vi "RollingCurrentReadout.vi"(4 "settling\ndelay":i32, 6 "Base/High Voltage?":enum16{"Base voltage", "High voltage"}(ring), 7 "Current Threshold [nA]":dbl, 8 "disabled channels IN":i32[](array[numeric]), 9 "Flag IN":i32[](array[numeric]), 10 "Current Array IN [nA]":dbl[](array[numeric])) -> (0 "disabled channels OUT":i32[](array[numeric]), 1 "Flag OUT":i32[](array[numeric]), 3 "Current Array OUT [nA]":dbl[](array[numeric]), 5 "Compliance exceeded":bool)   [LabVIEW 2013]
doc: "Switching through channels connected to a Probe Card"
uses:
  InstrControl/SupplyControl/SupplyControl.lvclass
  general_VIs/globals/QC_MeasurementSetup.vi
  InstrControl/InstrumentSetup.vi
  InstrControl/Switching/Switching.lvclass
  InstrControl/InstrControl.lvclass
panel:
  out "Display MUX":bool[][](array[boolean])
  out "Pinhole Flag":i32
  in  "last channel completed":i32
  # "Pickering Multiplexer Settings"
  # "X1"
  # "X2"
  # "X3"
  # "X4"
  # "X5"
  # "X6"
  # "X7"
  # "X8"
  # "Y1  Y2  Y3  Y4"
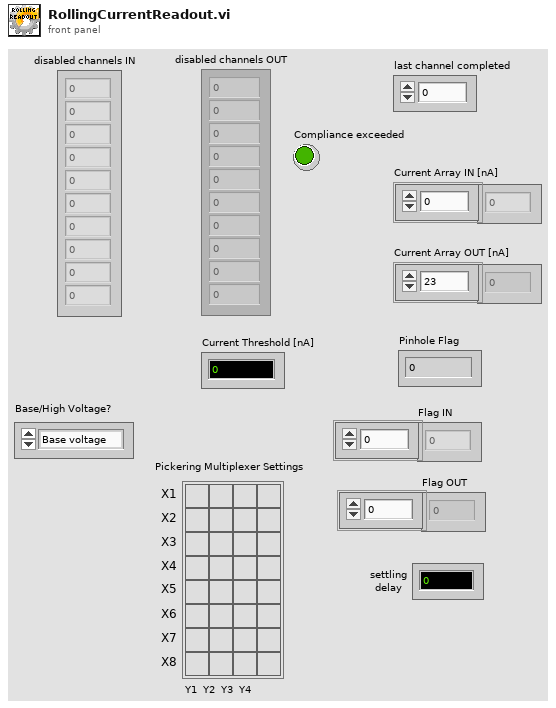
[diagram p1: front panel]
types:
  T1 = cluster{"Bias Supply":refnum<class "SupplyControl.lvclass">, "SMU":refnum<class "SupplyControl.lvclass">, "LCR":refnum<class "LCRControl.lvclass">, "Probe Card Channels":i32, "Bias Voltage [V]":dbl, "First strip":i32, "Last strip":i32, "Base Voltage [V]":dbl, "Base Ramp Step [V]":dbl, "Base Ramp Interval [ms]":u32, "High Voltage [V]":dbl, "High Ramp Step [V]":dbl, "High Ramp Interval [ms]":u32, "Single Needle":bool, "ArduinoControl.lvclass":refnum<class "ArduinoControl.lvclass">, "Fraction of good strips [%]":dbl}
  T2 = cluster{"GPIB address":string, "Matrix address":string, "Mux1 address":string, "Mux2 address":string, "Matrix used?":bool, "Switching":refnum<class "Switching.lvclass">, "Matrix X Channels":cluster{"Bias Supply / SMU LO":i32, "Bias Supply / SMU HI":i32, "CV Box LO":i32, "CV Box HI":i32, "CV Box LO IN":i32, "CV Box HI IN":i32, "Volt meter LO":i32, "Volt meter HI":i32, "Mux1 C1":i32, "Mux1 C2":i32, "Mux2 C1":i32, "Mux2 C2":i32}}
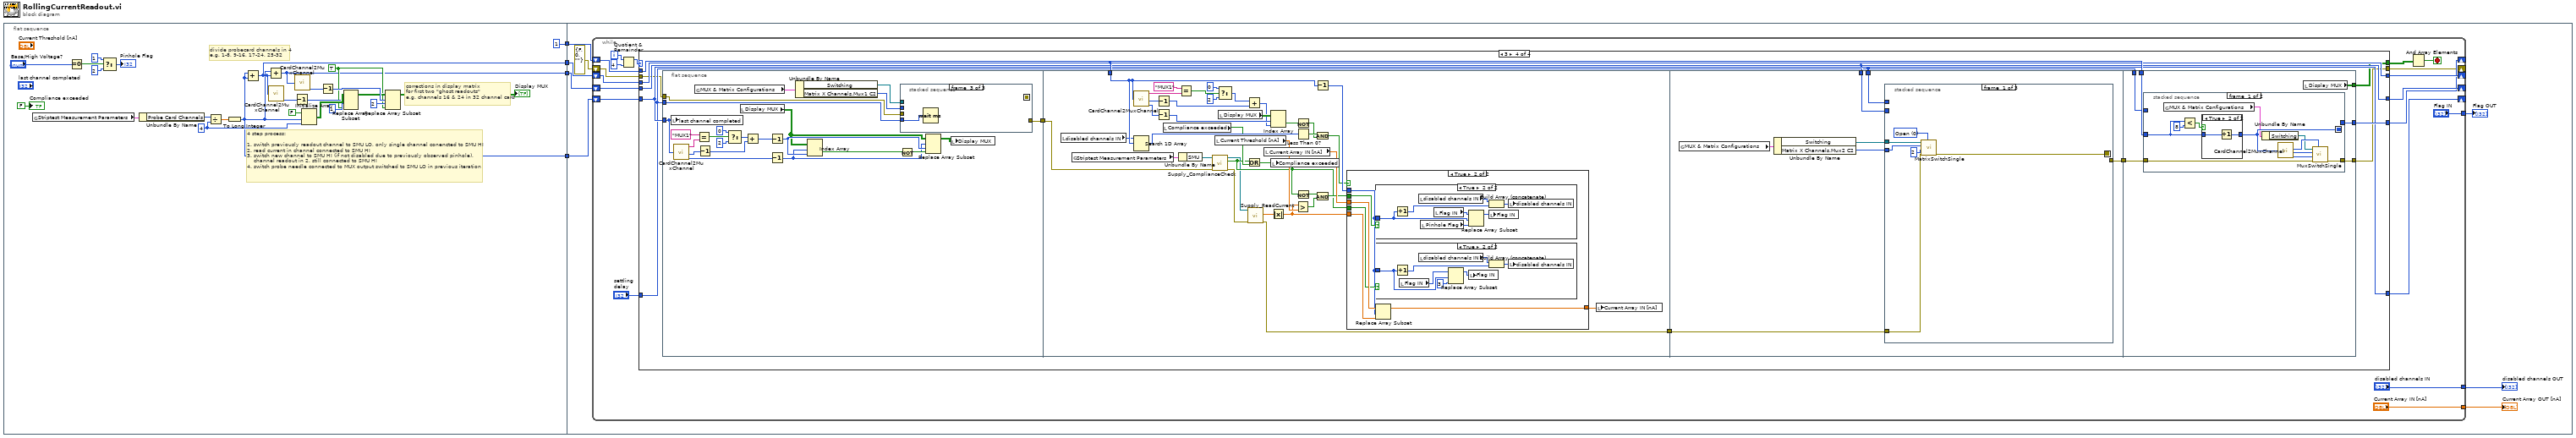
[diagram p0: block diagram]
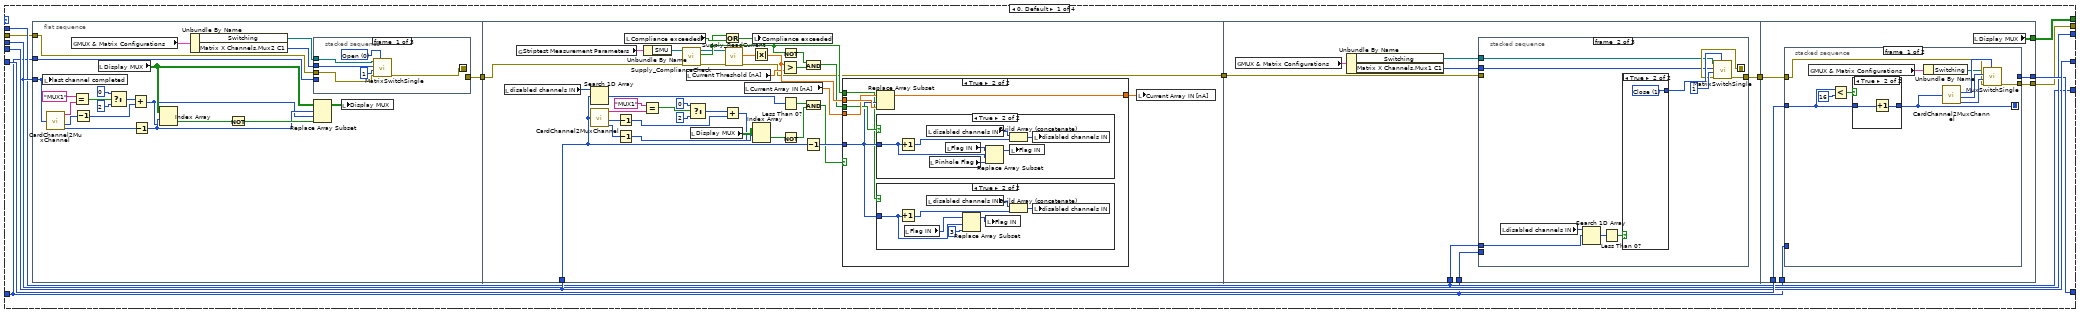
[diagram p2: hidden frame]
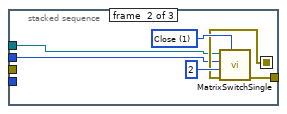
[diagram p3: hidden frame]
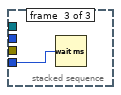
[diagram p4: hidden frame]
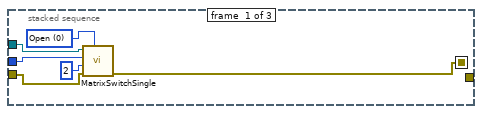
[diagram p8: hidden frame]
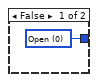
[diagram p9: hidden frame]
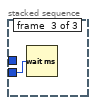
[diagram p10: hidden frame]
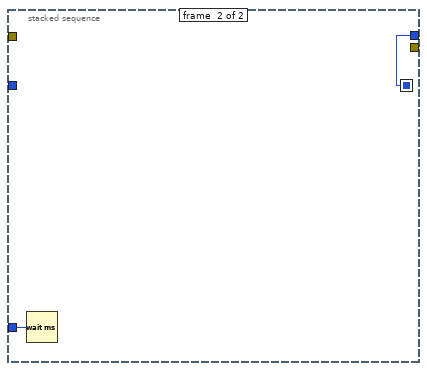
[diagram p12: hidden frame]
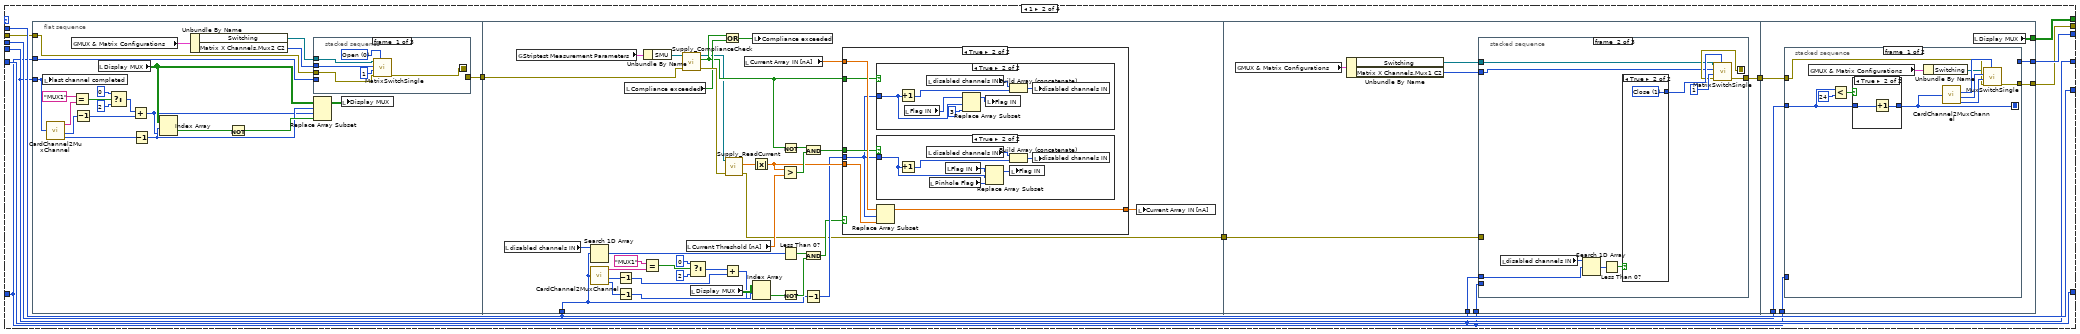
[diagram p13: hidden frame]
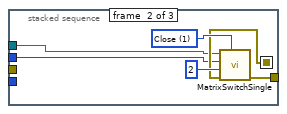
[diagram p14: hidden frame]
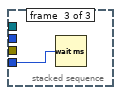
[diagram p15: hidden frame]
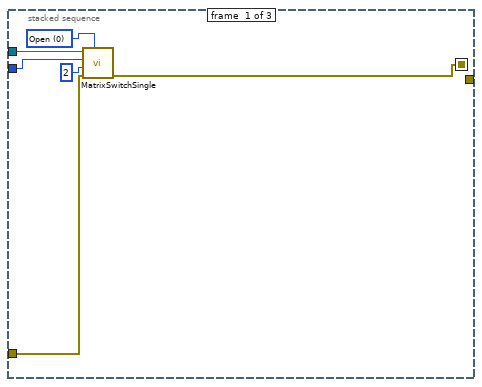
[diagram p19: hidden frame]
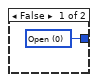
[diagram p20: hidden frame]
diagram:
  n1 = flat-sequence {
    tunnel: [1] -> w4
    tunnel: [w15] -> w3
    tunnel: [w14] -> w2
    tunnel: [w13] -> w1
    tunnel: w4 -> [w37]
    tunnel: w3 -> [w36]
    tunnel: w2 -> [w35]
    tunnel: w1 -> [w34]
    frame #0 {
      w17 = TRUE
      w27 = 4
      # "divide probecard channels in 4\ne.g. 1-8, 9-16, 17-24, 25-32"
      # "corrections in display matrix\nfor first two \"ghost readouts\"\ne.g. channels 16 & 24 in 32 channel card"
      # "4 step process:\n\n1. switch previously readout channel to SMU LO, only single channel conencted to SMU HI\n2. read current in channel connected to SMU HI\n3. switch new channel to SMU HI (if not disabled due to previously observed pinhole),\n    channel readout in 2. still connected to SMU HI\n4. switch probe needle connected to MUX output switched to SMU LO in previous iteration"
      n2 = global read "QC_MeasurementSetup.vi" "Striptest Measurement Parameters"() -> (w12:T1)
      n3 = Equal To 0?(x="Base/High Voltage?") -> (x = 0?=w7:bool)
      n4 = Select(t=1, s=w7, f=2) -> (s? t:f=→"Pinhole Flag":i32)
      n5 = Unbundle By Name(w12) -> ("Probe Card Channels"=w11:i32)
      n6 = Divide(x=w11, y=w27) -> (x/y=w29:dbl)
      n7 = To Long Integer(number=w29) -> (32bit integer=w15:i32)
      n8 = Add(x=w15, y=w15) -> (x+y=w13:i32)
      n9 = Add(x=w15, y=w13) -> (x+y=w14:i32)
      n10 = call "CardChannel2MuxChannel.vi"("Probecard Channel No."=w13) -> ("Channel"=w19:i32)  [unwired: 3 out]
      n11 = Decrement(x=w19) -> (x-1=w25:i32)
      n12 = call "CardChannel2MuxChannel.vi"("Probecard Channel No."=w14) -> ("Channel"=w18:i32)  [unwired: 3 out]
      n13 = Initialize Array(FALSE, w15, w27) -> (w26:bool[][])
      n14 = Decrement(x=w18) -> (x-1=w22:i32)
      n15 = Replace Array Subset(array=w26, new element=w17, index (row)=w25, index (col)=1) -> (w21:bool[][])
      n16 = Replace Array Subset(array=w21, new element=w17, index (row)=w22, index (col)=2) -> (→"Display MUX":bool[][])
      "Compliance exceeded" <- FALSE
    }
    frame #1 {
      n17 = while {
        shift-right: [w49] -> _
        shift-left: w35 -> [w52]
        shift-right: [w47] -> _
        shift-left: w34 -> [w50]
        shift-right: [w48] -> _
        shift-left: w36 -> [w51]
        shift-right: [w46] -> _
        shift-left: w37 -> [w56]
        tunnel: ["disabled channels IN"] -> w31
        tunnel: ["Current Array IN [nA]"] -> w32
        tunnel: ["Flag IN"] -> w33
        shift-right: [w39] -> _
        shift-left: errorcluster {"status"=FALSE, "code"=0, "source"=""} ("error constant") -> [w38]
        i -> [w53]
        stop <- w41 stop-if-true
        n18 = Quotient & Remainder(x=w53, y=4) -> (x-y*floor(x/y)=w54:i32)  [unwired: 1 out]
        n19 = case shown="3" w54 {
          tunnel: w56 -> [w64 w221 w374 w526]
          tunnel: w52 -> [w67 w218 w373 w523]
          tunnel: w51 -> [w68 w217 w371 w524]
          tunnel: w50 -> [w65 w219 w370 w525]
          tunnel: [w67 w218 w372 w523] -> w49
          tunnel: [w66 w217 w371 w524] -> w48
          tunnel: [w65 w220 w370 w525] -> w47
          tunnel: [w64 w221 w374 w527] -> w46
          tunnel: [w57 w210 w363 w516] -> w42
          tunnel: "settling\ndelay" -> [w63 w216 w369 w521]
          tunnel: [w61 w213 w366 w518] -> w39
          tunnel: w38 -> [w58 w211 w364 w517]
          frame 0, Default {
            n20 = flat-sequence {
              tunnel: w65 -> [w85]
              tunnel: w63 -> [w83]
              tunnel: [w82] -> w62
              tunnel: w58 -> [w81]
              tunnel: w67 -> [w105]
              tunnel: w62 -> [w118]
              tunnel: [w116] -> w59
              tunnel: w64 -> [w168]
              tunnel: w63 -> [w167]
              tunnel: [w166] -> w60
              tunnel: w59 -> [w165]
              tunnel: w68 -> [w193]
              tunnel: [w192] -> w66
              tunnel: w63 -> [w191]
              tunnel: [w190] -> w61
              tunnel: w60 -> [w189]
              tunnel: [w188] -> w57
              frame #0 {
                n21 = local write "last channel completed"(w85) -> ()
                n22 = call "CardChannel2MuxChannel.vi"("Probecard Channel No."=w85) -> ("Mux No. string"=w73:string, "C1 / C2"=w71:i32, "Channel"=w89:i32)  [unwired: 1 out]
                n23 = global read "InstrumentSetup.vi" "MUX & Matrix Configurations"() -> (w80:T2)
                n24 = Equal?(x="MUX1", y=w73) -> (x = y?=w76:bool)
                n25 = Decrement(x=w71) -> (x-1=w70:i32)
                n26 = local read "Display MUX"() -> (w90:bool[][])
                n27 = Select(t=0, s=w76, f=2) -> (s? t:f=w72:i32)
                n28 = Add(x=w72, y=w70) -> (x+y=w69:i32)
                n29 = Decrement(x=w89) -> (x-1=w86:i32)
                n30 = Index Array(array=w90, index (row)=w86, index (col)=w69) -> (element=w88:bool)
                n31 = Unbundle By Name(w80) -> ("Switching"=w79:refnum<class "Switching.lvclass">, "Matrix X Channels.Mux2 C1"=w78:i32)
                n32 = Not(x=w88) -> (.not. x?=w87:bool)
                n33 = stacked-sequence {
                  seq-local: [w94 _ _] -> [_ w100 _]
                  tunnel: [_ w99 _] -> w82
                  tunnel: w83 -> [_ _ w103]
                  tunnel: w81 -> [w93 _ _]
                  tunnel: w79 -> [w92 w98 _]
                  tunnel: w78 -> [w91 w97 _]
                  frame #0 {
                    w96 = u16 0 items=["Open", "Close"] ("Switch action")
                    n34 = call "MatrixSwitchSingle.vi"("Switch action"=w96, "error in (no error)"=w93, "Matrix Y"=1, "Matrix X"=w91, "Switching in"=w92) -> ("error out"=w94:errorcluster)  [unwired: 4 in, 2 out]
                  }
                  frame #1 {
                    w102 = u16 1 items=["Open", "Close"] ("Switch action")
                    n35 = call "MatrixSwitchSingle.vi"("Switch action"=w102, "error in (no error)"=w100, "Matrix Y"=2, "Matrix X"=w97, "Switching in"=w98) -> ("error out"=w99:errorcluster)  [unwired: 4 in, 2 out]
                  }
                  frame #2 {
                    n36 = Wait (ms)(milliseconds to wait=w103) -> ()  [unwired: 1 out]
                  }
                }
                n37 = Replace Array Subset(array=w90, new element=w87, index (row)=w86, index (col)=w69) -> (w84:bool[][])
                n38 = local write "Display MUX"(w84) -> ()
              }
              frame #1 {
                n39 = local read "disabled channels IN"() -> (w104:i32[])
                n40 = global read "QC_MeasurementSetup.vi" "Striptest Measurement Parameters"() -> (w120:T1)
                n41 = Search 1D Array(1D array=w104, element=w105) -> (index of element=w132:i32)  [unwired: 1 in]
                n42 = call "CardChannel2MuxChannel.vi"("Probecard Channel No."=w105) -> ("Mux No. string"=w108:string, "C1 / C2"=w109:i32, "Channel"=w107:i32)  [unwired: 1 out]
                n43 = Decrement(x=w109) -> (x-1=w110:i32)
                n44 = Decrement(x=w107) -> (x-1=w128:i32)
                n45 = local read "Compliance exceeded"() -> (w123:bool)
                n46 = Unbundle By Name(w120) -> ("SMU"=w119:refnum<class "SupplyControl.lvclass">)
                n47 = Equal?(x="MUX1", y=w108) -> (x = y?=w114:bool)
                n48 = call-dynamic "Supply_ComplianceCheck.vi"("error in (no error)"=w118, "SupplyControl in"=w119) -> ("error out"=w140:errorcluster, "Compliance exceeded?"=w122:bool, "SupplyControl out"=w117:refnum<class "SupplyControl.lvclass">)  [unwired: 6 in, 1 out]
                n49 = local read "Current Threshold [nA]"() -> (w135:dbl)
                n50 = Select(t=0, s=w114, f=2) -> (s? t:f=w111:i32)
                n51 = local read "Display MUX"() -> (w127:bool[][])
                n52 = Or(x=w122, y=w123) -> (x .or. y?=w121:bool)
                n53 = Add(x=w111, y=w110) -> (x+y=w106:i32)
                n54 = call-dynamic "Supply_ReadCurrent.vi"("error in (no error)"=w140, "SupplyControl in"=w117) -> ("error out"=w116:errorcluster, "Current in nA"=w137:dbl)  [unwired: 7 in, 1 out]
                n55 = local read "Current Array IN [nA]"() -> (w134:dbl[])
                n56 = local write "Compliance exceeded"(w121) -> ()
                n57 = Absolute Value(x=w137) -> (abs(x)=w136:dbl)
                n58 = Index Array(array=w127, index (row)=w128, index (col)=w106) -> (element=w129:bool)
                n59 = Greater?(x=w136, y=w135) -> (0:w138:bool)
                n60 = Not(x=w122) -> (.not. x?=w139:bool)
                n61 = Less Than 0?(x=w132) -> (x < 0?=w126:bool)
                n62 = Not(x=w129) -> (.not. x?=w125:bool)
                n63 = And(x=w139, y=w138) -> (x .and. y?=w130:bool)
                n64 = And(x=w126, y=w125) -> (x .and. y?=w124:bool)
                n65 = Decrement(x=w105) -> (x-1=w131:i32)
                n66 = case shown="True" w124 {
                  tunnel: w136 -> [_ w147]
                  tunnel: w134 -> [w141 w146]
                  tunnel: [w141 w145] -> w133
                  tunnel: w131 -> [_ w143]
                  tunnel: w130 -> [_ w144]
                  tunnel: w122 -> [_ w142]
                  frame False {
                  }
                  frame True {
                    n67 = Replace Array Subset(array=w146, new element=w147, index=w143) -> (w145:dbl[])
                    n68 = case shown="True" w144 {
                      tunnel: w143 -> [_ w158]
                      frame False {
                      }
                      frame True {
                        n69 = Increment(x=w158) -> (x+1=w157:i32)
                        n70 = local read "disabled channels IN"() -> (w159:i32[])
                        n71 = local read "Pinhole Flag"() -> (w155:i32)
                        n72 = local read "Flag IN"() -> (w161:i32[])
                        n73 = Replace Array Subset(array=w161, new element=w155, index=w158) -> (w160:i32[])
                        n74 = Build Array (concatenate)(w159, w157) -> (w156:i32[])
                        n75 = local write "Flag IN"(w160) -> ()
                        n76 = local write "disabled channels IN"(w156) -> ()
                      }
                    }
                    n77 = case shown="True" w142 {
                      tunnel: w143 -> [_ w148]
                      frame False {
                      }
                      frame True {
                        n78 = Increment(x=w148) -> (x+1=w149:i32)
                        n79 = local read "Flag IN"() -> (w153:i32[])
                        n80 = local read "disabled channels IN"() -> (w151:i32[])
                        n81 = Replace Array Subset(array=w153, new element=3, index=w148) -> (w152:i32[])
                        n82 = local write "Flag IN"(w152) -> ()
                        n83 = Build Array (concatenate)(w151, w149) -> (w150:i32[])
                        n84 = local write "disabled channels IN"(w150) -> ()
                      }
                    }
                  }
                }
                n85 = local write "Current Array IN [nA]"(w133) -> ()
              }
              frame #2 {
                n86 = global read "InstrumentSetup.vi" "MUX & Matrix Configurations"() -> (w164:T2)
                n87 = Unbundle By Name(w164) -> ("Switching"=w163:refnum<class "Switching.lvclass">, "Matrix X Channels.Mux1 C1"=w162:i32)
                n88 = stacked-sequence {
                  seq-local: [w172 _ _] -> [_ w178 _]
                  tunnel: w168 -> [_ w180 _]
                  tunnel: [_ w179 _] -> w166
                  tunnel: w167 -> [_ _ w187]
                  tunnel: w165 -> [w171 _ _]
                  tunnel: w163 -> [w170 w177 _]
                  tunnel: w162 -> [w169 w176 _]
                  frame #0 {
                    w173 = u16 0 items=["Open", "Close"] ("Switch action")
                    n89 = call "MatrixSwitchSingle.vi"("Switch action"=w173, "error in (no error)"=w171, "Matrix Y"=2, "Matrix X"=w169, "Switching in"=w170) -> ("error out"=w172:errorcluster)  [unwired: 4 in, 2 out]
                  }
                  frame #1 {
                    n90 = local read "disabled channels IN"() -> (w175:i32[])
                    n91 = Search 1D Array(1D array=w175, element=w180) -> (index of element=w182:i32)  [unwired: 1 in]
                    n92 = Less Than 0?(x=w182) -> (x < 0?=w183:bool)
                    n93 = case shown="True" w183 {
                      tunnel: [w185 w186] -> w181
                      frame False {
                        w185 = u16 0 items=["Open", "Close"] ("Switch action")
                      }
                      frame True {
                        w186 = u16 1 items=["Open", "Close"] ("Switch action")
                      }
                    }
                    n94 = call "MatrixSwitchSingle.vi"("Switch action"=w181, "error in (no error)"=w178, "Matrix Y"=1, "Matrix X"=w176, "Switching in"=w177) -> ("error out"=w179:errorcluster)  [unwired: 4 in, 2 out]
                  }
                  frame #2 {
                    n95 = Wait (ms)(milliseconds to wait=w187) -> ()  [unwired: 1 out]
                  }
                }
              }
              frame #3 {
                n96 = stacked-sequence {
                  seq-local: [w198 _] -> [_ w209]
                  tunnel: w193 -> [w200 _]
                  tunnel: [w197 _] -> w190
                  tunnel: w189 -> [w196 _]
                  tunnel: [_ w209] -> w192
                  tunnel: w191 -> [_ w208]
                  frame #0 {
                    n97 = global read "InstrumentSetup.vi" "MUX & Matrix Configurations"() -> (w195:T2)
                    n98 = Less?(x=w200, y=16) -> (x < y?=w201:bool)
                    n99 = case shown="True" w201 {
                      tunnel: w200 -> [w205 w207]
                      tunnel: [w205 w206] -> w198
                      frame False {
                      }
                      frame True {
                        n100 = Increment(x=w207) -> (x+1=w206:i32)
                      }
                    }
                    n101 = Unbundle By Name(w195) -> ("Switching"=w194:refnum<class "Switching.lvclass">)
                    n102 = call "CardChannel2MuxChannel.vi"("Probecard Channel No."=w198) -> ("Mux No.:"=w202:u32, "C1 / C2"=w203:i32, "Channel"=w204:i32)  [unwired: 1 out]
                    n103 = call "MuxSwitchSingle.vi"("MUX address"=w202, "error in (no error)"=w196, "Channel"=w204, "C1 / C2"=w203, "Switching in"=w194) -> ("error out"=w197:errorcluster)  [unwired: 4 in, 2 out]
                  }
                  frame #1 {
                    n104 = Wait (ms)(milliseconds to wait=w208) -> ()  [unwired: 1 out]
                  }
                }
                n105 = local read "Display MUX"() -> (w188:bool[][])
              }
            }
          }
          frame 1 {
            n106 = flat-sequence {
              tunnel: w218 -> [w238]
              tunnel: w216 -> [w236]
              tunnel: [w235] -> w215
              tunnel: w211 -> [w234]
              tunnel: w221 -> [w258]
              tunnel: w215 -> [w271]
              tunnel: [w269] -> w212
              tunnel: w217 -> [w321]
              tunnel: w216 -> [w320]
              tunnel: [w319] -> w214
              tunnel: w212 -> [w318]
              tunnel: w219 -> [w346]
              tunnel: [w345] -> w220
              tunnel: w216 -> [w344]
              tunnel: w214 -> [w343]
              tunnel: [w342] -> w213
              tunnel: [w341] -> w210
              frame #0 {
                n107 = local write "last channel completed"(w238) -> ()
                n108 = call "CardChannel2MuxChannel.vi"("Probecard Channel No."=w238) -> ("Mux No. string"=w224:string, "C1 / C2"=w222:i32, "Channel"=w242:i32)  [unwired: 1 out]
                n109 = global read "InstrumentSetup.vi" "MUX & Matrix Configurations"() -> (w233:T2)
                n110 = Equal?(x="MUX1", y=w224) -> (x = y?=w229:bool)
                n111 = Decrement(x=w222) -> (x-1=w225:i32)
                n112 = local read "Display MUX"() -> (w243:bool[][])
                n113 = Select(t=0, s=w229, f=2) -> (s? t:f=w226:i32)
                n114 = Add(x=w226, y=w225) -> (x+y=w223:i32)
                n115 = Decrement(x=w242) -> (x-1=w239:i32)
                n116 = Index Array(array=w243, index (row)=w239, index (col)=w223) -> (element=w241:bool)
                n117 = Unbundle By Name(w233) -> ("Switching"=w232:refnum<class "Switching.lvclass">, "Matrix X Channels.Mux2 C2"=w231:i32)
                n118 = Not(x=w241) -> (.not. x?=w240:bool)
                n119 = stacked-sequence {
                  seq-local: [w247 _ _] -> [_ w253 _]
                  tunnel: [_ w252 _] -> w235
                  tunnel: w236 -> [_ _ w256]
                  tunnel: w234 -> [w246 _ _]
                  tunnel: w232 -> [w245 w250 _]
                  tunnel: w231 -> [w244 w251 _]
                  frame #0 {
                    w249 = u16 0 items=["Open", "Close"] ("Switch action")
                    n120 = call "MatrixSwitchSingle.vi"("Switch action"=w249, "error in (no error)"=w246, "Matrix Y"=1, "Matrix X"=w244, "Switching in"=w245) -> ("error out"=w247:errorcluster)  [unwired: 4 in, 2 out]
                  }
                  frame #1 {
                    w255 = u16 1 items=["Open", "Close"] ("Switch action")
                    n121 = call "MatrixSwitchSingle.vi"("Switch action"=w255, "error in (no error)"=w253, "Matrix Y"=2, "Matrix X"=w251, "Switching in"=w250) -> ("error out"=w252:errorcluster)  [unwired: 4 in, 2 out]
                  }
                  frame #2 {
                    n122 = Wait (ms)(milliseconds to wait=w256) -> ()  [unwired: 1 out]
                  }
                }
                n123 = Replace Array Subset(array=w243, new element=w240, index (row)=w239, index (col)=w223) -> (w237:bool[][])
                n124 = local write "Display MUX"(w237) -> ()
              }
              frame #1 {
                n125 = local read "disabled channels IN"() -> (w257:i32[])
                n126 = global read "QC_MeasurementSetup.vi" "Striptest Measurement Parameters"() -> (w273:T1)
                n127 = Search 1D Array(1D array=w257, element=w258) -> (index of element=w285:i32)  [unwired: 1 in]
                n128 = call "CardChannel2MuxChannel.vi"("Probecard Channel No."=w258) -> ("Mux No. string"=w261:string, "C1 / C2"=w262:i32, "Channel"=w260:i32)  [unwired: 1 out]
                n129 = Decrement(x=w262) -> (x-1=w263:i32)
                n130 = Decrement(x=w260) -> (x-1=w281:i32)
                n131 = local read "Compliance exceeded"() -> (w276:bool)
                n132 = Unbundle By Name(w273) -> ("SMU"=w272:refnum<class "SupplyControl.lvclass">)
                n133 = Equal?(x="MUX1", y=w261) -> (x = y?=w267:bool)
                n134 = call-dynamic "Supply_ComplianceCheck.vi"("error in (no error)"=w271, "SupplyControl in"=w272) -> ("error out"=w293:errorcluster, "Compliance exceeded?"=w274:bool, "SupplyControl out"=w270:refnum<class "SupplyControl.lvclass">)  [unwired: 6 in, 1 out]
                n135 = local read "Current Threshold [nA]"() -> (w289:dbl)
                n136 = Select(t=0, s=w267, f=2) -> (s? t:f=w264:i32)
                n137 = local read "Display MUX"() -> (w280:bool[][])
                n138 = Or(x=w274, y=w276) -> (x .or. y?=w275:bool)
                n139 = Add(x=w264, y=w263) -> (x+y=w259:i32)
                n140 = call-dynamic "Supply_ReadCurrent.vi"("error in (no error)"=w293, "SupplyControl in"=w270) -> ("error out"=w269:errorcluster, "Current in nA"=w290:dbl)  [unwired: 7 in, 1 out]
                n141 = local read "Current Array IN [nA]"() -> (w288:dbl[])
                n142 = local write "Compliance exceeded"(w275) -> ()
                n143 = Absolute Value(x=w290) -> (abs(x)=w286:dbl)
                n144 = Index Array(array=w280, index (row)=w281, index (col)=w259) -> (element=w282:bool)
                n145 = Greater?(x=w286, y=w289) -> (0:w291:bool)
                n146 = Not(x=w274) -> (.not. x?=w292:bool)
                n147 = Less Than 0?(x=w285) -> (x < 0?=w279:bool)
                n148 = Not(x=w282) -> (.not. x?=w278:bool)
                n149 = And(x=w292, y=w291) -> (x .and. y?=w283:bool)
                n150 = And(x=w279, y=w278) -> (x .and. y?=w277:bool)
                n151 = Decrement(x=w258) -> (x-1=w284:i32)
                n152 = case shown="True" w277 {
                  tunnel: w288 -> [w294 w300]
                  tunnel: [w294 w299] -> w287
                  tunnel: w284 -> [_ w296]
                  tunnel: w286 -> [_ w298]
                  tunnel: w283 -> [_ w297]
                  tunnel: w274 -> [_ w295]
                  frame False {
                  }
                  frame True {
                    n153 = case shown="True" w295 {
                      tunnel: w296 -> [_ w301]
                      frame False {
                      }
                      frame True {
                        n154 = Increment(x=w301) -> (x+1=w302:i32)
                        n155 = local read "Flag IN"() -> (w306:i32[])
                        n156 = local read "disabled channels IN"() -> (w304:i32[])
                        n157 = Replace Array Subset(array=w306, new element=3, index=w301) -> (w305:i32[])
                        n158 = local write "Flag IN"(w305) -> ()
                        n159 = Build Array (concatenate)(w304, w302) -> (w303:i32[])
                        n160 = local write "disabled channels IN"(w303) -> ()
                      }
                    }
                    n161 = case shown="True" w297 {
                      tunnel: w296 -> [_ w311]
                      frame False {
                      }
                      frame True {
                        n162 = Increment(x=w311) -> (x+1=w310:i32)
                        n163 = local read "disabled channels IN"() -> (w312:i32[])
                        n164 = local read "Pinhole Flag"() -> (w308:i32)
                        n165 = local read "Flag IN"() -> (w314:i32[])
                        n166 = Replace Array Subset(array=w314, new element=w308, index=w311) -> (w313:i32[])
                        n167 = Build Array (concatenate)(w312, w310) -> (w309:i32[])
                        n168 = local write "Flag IN"(w313) -> ()
                        n169 = local write "disabled channels IN"(w309) -> ()
                      }
                    }
                    n170 = Replace Array Subset(array=w300, new element=w298, index=w296) -> (w299:dbl[])
                  }
                }
                n171 = local write "Current Array IN [nA]"(w287) -> ()
              }
              frame #2 {
                n172 = global read "InstrumentSetup.vi" "MUX & Matrix Configurations"() -> (w317:T2)
                n173 = Unbundle By Name(w317) -> ("Switching"=w316:refnum<class "Switching.lvclass">, "Matrix X Channels.Mux1 C2"=w315:i32)
                n174 = stacked-sequence {
                  seq-local: [w325 _ _] -> [_ w332 _]
                  tunnel: w321 -> [_ w333 _]
                  tunnel: [_ w331 _] -> w319
                  tunnel: w320 -> [_ _ w340]
                  tunnel: w318 -> [w324 _ _]
                  tunnel: w316 -> [w323 w330 _]
                  tunnel: w315 -> [w322 w329 _]
                  frame #0 {
                    w326 = u16 0 items=["Open", "Close"] ("Switch action")
                    n175 = call "MatrixSwitchSingle.vi"("Switch action"=w326, "error in (no error)"=w324, "Matrix Y"=2, "Matrix X"=w322, "Switching in"=w323) -> ("error out"=w325:errorcluster)  [unwired: 4 in, 2 out]
                  }
                  frame #1 {
                    n176 = local read "disabled channels IN"() -> (w328:i32[])
                    n177 = Search 1D Array(1D array=w328, element=w333) -> (index of element=w334:i32)  [unwired: 1 in]
                    n178 = Less Than 0?(x=w334) -> (x < 0?=w335:bool)
                    n179 = case shown="True" w335 {
                      tunnel: [w338 w339] -> w336
                      frame False {
                        w338 = u16 0 items=["Open", "Close"] ("Switch action")
                      }
                      frame True {
                        w339 = u16 1 items=["Open", "Close"] ("Switch action")
                      }
                    }
                    n180 = call "MatrixSwitchSingle.vi"("Switch action"=w336, "error in (no error)"=w332, "Matrix Y"=1, "Matrix X"=w329, "Switching in"=w330) -> ("error out"=w331:errorcluster)  [unwired: 4 in, 2 out]
                  }
                  frame #2 {
                    n181 = Wait (ms)(milliseconds to wait=w340) -> ()  [unwired: 1 out]
                  }
                }
              }
              frame #3 {
                n182 = stacked-sequence {
                  seq-local: [w351 _] -> [_ w362]
                  tunnel: w346 -> [w352 _]
                  tunnel: w343 -> [w350 _]
                  tunnel: [_ w362] -> w345
                  tunnel: w344 -> [_ w361]
                  tunnel: [w347 _] -> w342
                  frame #0 {
                    n183 = global read "InstrumentSetup.vi" "MUX & Matrix Configurations"() -> (w349:T2)
                    n184 = Less?(x=w352, y=24) -> (x < y?=w354:bool)
                    n185 = case shown="True" w354 {
                      tunnel: w352 -> [w358 w360]
                      tunnel: [w358 w359] -> w351
                      frame False {
                      }
                      frame True {
                        n186 = Increment(x=w360) -> (x+1=w359:i32)
                      }
                    }
                    n187 = Unbundle By Name(w349) -> ("Switching"=w348:refnum<class "Switching.lvclass">)
                    n188 = call "CardChannel2MuxChannel.vi"("Probecard Channel No."=w351) -> ("Mux No.:"=w355:u32, "C1 / C2"=w356:i32, "Channel"=w357:i32)  [unwired: 1 out]
                    n189 = call "MuxSwitchSingle.vi"("MUX address"=w355, "error in (no error)"=w350, "Channel"=w357, "C1 / C2"=w356, "Switching in"=w348) -> ("error out"=w347:errorcluster)  [unwired: 4 in, 2 out]
                  }
                  frame #1 {
                    n190 = Wait (ms)(milliseconds to wait=w361) -> ()  [unwired: 1 out]
                  }
                }
                n191 = local read "Display MUX"() -> (w341:bool[][])
              }
            }
          }
          frame 2 {
            n192 = flat-sequence {
              tunnel: w374 -> [w396]
              tunnel: w369 -> [w389]
              tunnel: [w388] -> w368
              tunnel: w364 -> [w387]
              tunnel: w371 -> [w411]
              tunnel: w368 -> [w424]
              tunnel: [w422] -> w365
              tunnel: w370 -> [w474]
              tunnel: w369 -> [w473]
              tunnel: [w472] -> w367
              tunnel: w365 -> [w471]
              tunnel: w373 -> [w499]
              tunnel: [w498] -> w372
              tunnel: w369 -> [w497]
              tunnel: w367 -> [w496]
              tunnel: [w495] -> w366
              tunnel: [w494] -> w363
              frame #0 {
                n193 = local write "last channel completed"(w396) -> ()
                n194 = call "CardChannel2MuxChannel.vi"("Probecard Channel No."=w396) -> ("Mux No. string"=w376:string, "C1 / C2"=w377:i32, "Channel"=w395:i32)  [unwired: 1 out]
                n195 = global read "InstrumentSetup.vi" "MUX & Matrix Configurations"() -> (w386:T2)
                n196 = Equal?(x="MUX1", y=w376) -> (x = y?=w382:bool)
                n197 = Decrement(x=w377) -> (x-1=w378:i32)
                n198 = local read "Display MUX"() -> (w392:bool[][])
                n199 = Select(t=0, s=w382, f=2) -> (s? t:f=w379:i32)
                n200 = Add(x=w379, y=w378) -> (x+y=w375:i32)
                n201 = Decrement(x=w395) -> (x-1=w391:i32)
                n202 = Index Array(array=w392, index (row)=w391, index (col)=w375) -> (element=w394:bool)
                n203 = Unbundle By Name(w386) -> ("Switching"=w385:refnum<class "Switching.lvclass">, "Matrix X Channels.Mux1 C1"=w384:i32)
                n204 = Not(x=w394) -> (.not. x?=w393:bool)
                n205 = Replace Array Subset(array=w392, new element=w393, index (row)=w391, index (col)=w375) -> (w390:bool[][])
                n206 = stacked-sequence {
                  seq-local: [w400 _ _] -> [_ w406 _]
                  tunnel: w387 -> [w399 _ _]
                  tunnel: [_ w405 _] -> w388
                  tunnel: w389 -> [_ _ w409]
                  tunnel: w385 -> [w398 w404 _]
                  tunnel: w384 -> [w397 w403 _]
                  frame #0 {
                    w402 = u16 0 items=["Open", "Close"] ("Switch action")
                    n207 = call "MatrixSwitchSingle.vi"("Switch action"=w402, "error in (no error)"=w399, "Matrix Y"=1, "Matrix X"=w397, "Switching in"=w398) -> ("error out"=w400:errorcluster)  [unwired: 4 in, 2 out]
                  }
                  frame #1 {
                    w408 = u16 1 items=["Open", "Close"] ("Switch action")
                    n208 = call "MatrixSwitchSingle.vi"("Switch action"=w408, "error in (no error)"=w406, "Matrix Y"=2, "Matrix X"=w403, "Switching in"=w404) -> ("error out"=w405:errorcluster)  [unwired: 4 in, 2 out]
                  }
                  frame #2 {
                    n209 = Wait (ms)(milliseconds to wait=w409) -> ()  [unwired: 1 out]
                  }
                }
                n210 = local write "Display MUX"(w390) -> ()
              }
              frame #1 {
                n211 = local read "disabled channels IN"() -> (w410:i32[])
                n212 = global read "QC_MeasurementSetup.vi" "Striptest Measurement Parameters"() -> (w426:T1)
                n213 = Search 1D Array(1D array=w410, element=w411) -> (index of element=w438:i32)  [unwired: 1 in]
                n214 = call "CardChannel2MuxChannel.vi"("Probecard Channel No."=w411) -> ("Mux No. string"=w414:string, "C1 / C2"=w415:i32, "Channel"=w412:i32)  [unwired: 1 out]
                n215 = Decrement(x=w415) -> (x-1=w416:i32)
                n216 = Decrement(x=w412) -> (x-1=w435:i32)
                n217 = local read "Compliance exceeded"() -> (w429:bool)
                n218 = Unbundle By Name(w426) -> ("SMU"=w425:refnum<class "SupplyControl.lvclass">)
                n219 = Equal?(x="MUX1", y=w414) -> (x = y?=w420:bool)
                n220 = call-dynamic "Supply_ComplianceCheck.vi"("error in (no error)"=w424, "SupplyControl in"=w425) -> ("error out"=w446:errorcluster, "Compliance exceeded?"=w428:bool, "SupplyControl out"=w423:refnum<class "SupplyControl.lvclass">)  [unwired: 6 in, 1 out]
                n221 = local read "Current Threshold [nA]"() -> (w442:dbl)
                n222 = Select(t=0, s=w420, f=2) -> (s? t:f=w417:i32)
                n223 = local read "Display MUX"() -> (w434:bool[][])
                n224 = Or(x=w428, y=w429) -> (x .or. y?=w427:bool)
                n225 = Add(x=w417, y=w416) -> (x+y=w413:i32)
                n226 = call-dynamic "Supply_ReadCurrent.vi"("error in (no error)"=w446, "SupplyControl in"=w423) -> ("error out"=w422:errorcluster, "Current in nA"=w443:dbl)  [unwired: 7 in, 1 out]
                n227 = local read "Current Array IN [nA]"() -> (w441:dbl[])
                n228 = local write "Compliance exceeded"(w427) -> ()
                n229 = Absolute Value(x=w443) -> (abs(x)=w439:dbl)
                n230 = Index Array(array=w434, index (row)=w435, index (col)=w413) -> (element=w431:bool)
                n231 = Greater?(x=w439, y=w442) -> (0:w444:bool)
                n232 = Not(x=w428) -> (.not. x?=w445:bool)
                n233 = Less Than 0?(x=w438) -> (x < 0?=w433:bool)
                n234 = Not(x=w431) -> (.not. x?=w430:bool)
                n235 = And(x=w445, y=w444) -> (x .and. y?=w436:bool)
                n236 = And(x=w433, y=w430) -> (x .and. y?=w432:bool)
                n237 = Decrement(x=w411) -> (x-1=w437:i32)
                n238 = case shown="True" w432 {
                  tunnel: w439 -> [_ w453]
                  tunnel: w441 -> [w447 w452]
                  tunnel: [w447 w451] -> w440
                  tunnel: w437 -> [_ w449]
                  tunnel: w428 -> [_ w450]
                  tunnel: w436 -> [_ w448]
                  frame False {
                  }
                  frame True {
                    n239 = Replace Array Subset(array=w452, new element=w453, index=w449) -> (w451:dbl[])
                    n240 = case shown="True" w448 {
                      tunnel: w449 -> [_ w457]
                      frame False {
                      }
                      frame True {
                        n241 = Increment(x=w457) -> (x+1=w456:i32)
                        n242 = local read "disabled channels IN"() -> (w458:i32[])
                        n243 = local read "Pinhole Flag"() -> (w454:i32)
                        n244 = local read "Flag IN"() -> (w460:i32[])
                        n245 = Replace Array Subset(array=w460, new element=w454, index=w457) -> (w459:i32[])
                        n246 = Build Array (concatenate)(w458, w456) -> (w455:i32[])
                        n247 = local write "Flag IN"(w459) -> ()
                        n248 = local write "disabled channels IN"(w455) -> ()
                      }
                    }
                    n249 = case shown="True" w450 {
                      tunnel: w449 -> [_ w461]
                      frame False {
                      }
                      frame True {
                        n250 = Increment(x=w461) -> (x+1=w462:i32)
                        n251 = local read "Flag IN"() -> (w466:i32[])
                        n252 = local read "disabled channels IN"() -> (w464:i32[])
                        n253 = Replace Array Subset(array=w466, new element=3, index=w461) -> (w465:i32[])
                        n254 = local write "Flag IN"(w465) -> ()
                        n255 = Build Array (concatenate)(w464, w462) -> (w463:i32[])
                        n256 = local write "disabled channels IN"(w463) -> ()
                      }
                    }
                  }
                }
                n257 = local write "Current Array IN [nA]"(w440) -> ()
              }
              frame #2 {
                n258 = global read "InstrumentSetup.vi" "MUX & Matrix Configurations"() -> (w470:T2)
                n259 = Unbundle By Name(w470) -> ("Switching"=w469:refnum<class "Switching.lvclass">, "Matrix X Channels.Mux2 C1"=w468:i32)
                n260 = stacked-sequence {
                  seq-local: [w478 _ _] -> [_ w484 _]
                  tunnel: w471 -> [w477 _ _]
                  tunnel: w474 -> [_ w486 _]
                  tunnel: [_ w485 _] -> w472
                  tunnel: w473 -> [_ _ w493]
                  tunnel: w469 -> [w476 w483 _]
                  tunnel: w468 -> [w475 w482 _]
                  frame #0 {
                    w479 = u16 0 items=["Open", "Close"] ("Switch action")
                    n261 = call "MatrixSwitchSingle.vi"("Switch action"=w479, "error in (no error)"=w477, "Matrix Y"=2, "Matrix X"=w475, "Switching in"=w476) -> ("error out"=w478:errorcluster)  [unwired: 4 in, 2 out]
                  }
                  frame #1 {
                    n262 = local read "disabled channels IN"() -> (w481:i32[])
                    n263 = Search 1D Array(1D array=w481, element=w486) -> (index of element=w488:i32)  [unwired: 1 in]
                    n264 = Less Than 0?(x=w488) -> (x < 0?=w489:bool)
                    n265 = case shown="True" w489 {
                      tunnel: [w491 w492] -> w487
                      frame False {
                        w491 = u16 0 items=["Open", "Close"] ("Switch action")
                      }
                      frame True {
                        w492 = u16 1 items=["Open", "Close"] ("Switch action")
                      }
                    }
                    n266 = call "MatrixSwitchSingle.vi"("Switch action"=w487, "error in (no error)"=w484, "Matrix Y"=1, "Matrix X"=w482, "Switching in"=w483) -> ("error out"=w485:errorcluster)  [unwired: 4 in, 2 out]
                  }
                  frame #2 {
                    n267 = Wait (ms)(milliseconds to wait=w493) -> ()  [unwired: 1 out]
                  }
                }
              }
              frame #3 {
                n268 = stacked-sequence {
                  seq-local: [w504 _] -> [_ w515]
                  tunnel: w499 -> [w505 _]
                  tunnel: w496 -> [w503 _]
                  tunnel: [w502 _] -> w495
                  tunnel: [_ w515] -> w498
                  tunnel: w497 -> [_ w514]
                  frame #0 {
                    n269 = global read "InstrumentSetup.vi" "MUX & Matrix Configurations"() -> (w501:T2)
                    n270 = Less?(x=w505, y=32) -> (x < y?=w507:bool)
                    n271 = case shown="True" w507 {
                      tunnel: w505 -> [w511 w513]
                      tunnel: [w511 w512] -> w504
                      frame False {
                      }
                      frame True {
                        n272 = Increment(x=w513) -> (x+1=w512:i32)
                      }
                    }
                    n273 = Unbundle By Name(w501) -> ("Switching"=w500:refnum<class "Switching.lvclass">)
                    n274 = call "CardChannel2MuxChannel.vi"("Probecard Channel No."=w504) -> ("Mux No.:"=w508:u32, "C1 / C2"=w509:i32, "Channel"=w510:i32)  [unwired: 1 out]
                    n275 = call "MuxSwitchSingle.vi"("MUX address"=w508, "error in (no error)"=w503, "Channel"=w510, "C1 / C2"=w509, "Switching in"=w500) -> ("error out"=w502:errorcluster)  [unwired: 4 in, 2 out]
                  }
                  frame #1 {
                    n276 = Wait (ms)(milliseconds to wait=w514) -> ()  [unwired: 1 out]
                  }
                }
                n277 = local read "Display MUX"() -> (w494:bool[][])
              }
            }
          }
          frame 3 {
            n278 = flat-sequence {
              tunnel: w524 -> [w545]
              tunnel: w521 -> [w542]
              tunnel: [w541] -> w522
              tunnel: w517 -> [w540]
              tunnel: w525 -> [w567]
              tunnel: w522 -> [w580]
              tunnel: [w576] -> w520
              tunnel: w523 -> [w628]
              tunnel: w521 -> [w627]
              tunnel: w520 -> [w626]
              tunnel: [w625] -> w519
              tunnel: w526 -> [w653]
              tunnel: [w652] -> w527
              tunnel: w521 -> [w651]
              tunnel: w519 -> [w650]
              tunnel: [w649] -> w518
              tunnel: [w648] -> w516
              frame #0 {
                n279 = local write "last channel completed"(w545) -> ()
                n280 = call "CardChannel2MuxChannel.vi"("Probecard Channel No."=w545) -> ("Mux No. string"=w528:string, "C1 / C2"=w530:i32, "Channel"=w550:i32)  [unwired: 1 out]
                n281 = global read "InstrumentSetup.vi" "MUX & Matrix Configurations"() -> (w539:T2)
                n282 = Equal?(x="MUX1", y=w528) -> (x = y?=w535:bool)
                n283 = Decrement(x=w530) -> (x-1=w531:i32)
                n284 = Select(t=0, s=w535, f=2) -> (s? t:f=w532:i32)
                n285 = local read "Display MUX"() -> (w544:bool[][])
                n286 = Add(x=w532, y=w531) -> (x+y=w529:i32)
                n287 = Decrement(x=w529) -> (x-1=w547:i32)
                n288 = Decrement(x=w550) -> (x-1=w546:i32)
                n289 = Unbundle By Name(w539) -> ("Switching"=w538:refnum<class "Switching.lvclass">, "Matrix X Channels.Mux1 C2"=w537:i32)
                n290 = Index Array(array=w544, index (row)=w546, index (col)=w547) -> (element=w549:bool)
                n291 = Not(x=w549) -> (.not. x?=w548:bool)
                n292 = stacked-sequence {
                  seq-local: [w554 _ _] -> [_ w560 _]
                  tunnel: [_ w559 _] -> w541
                  tunnel: w542 -> [_ _ w563]
                  tunnel: w540 -> [w553 _ _]
                  tunnel: w538 -> [w552 w557 _]
                  tunnel: w537 -> [w551 w558 _]
                  frame #0 {
                    w556 = u16 0 items=["Open", "Close"] ("Switch action")
                    n293 = call "MatrixSwitchSingle.vi"("Switch action"=w556, "error in (no error)"=w553, "Matrix Y"=1, "Matrix X"=w551, "Switching in"=w552) -> ("error out"=w554:errorcluster)  [unwired: 4 in, 2 out]
                  }
                  frame #1 {
                    w562 = u16 1 items=["Open", "Close"] ("Switch action")
                    n294 = call "MatrixSwitchSingle.vi"("Switch action"=w562, "error in (no error)"=w560, "Matrix Y"=2, "Matrix X"=w558, "Switching in"=w557) -> ("error out"=w559:errorcluster)  [unwired: 4 in, 2 out]
                  }
                  frame #2 {
                    n295 = Wait (ms)(milliseconds to wait=w563) -> ()  [unwired: 1 out]
                  }
                }
                n296 = Replace Array Subset(array=w544, new element=w548, index (row)=w546, index (col)=w547) -> (w543:bool[][])
                n297 = local write "Display MUX"(w543) -> ()
              }
              frame #1 {
                n298 = local read "disabled channels IN"() -> (w564:i32[])
                n299 = global read "QC_MeasurementSetup.vi" "Striptest Measurement Parameters"() -> (w578:T1)
                n300 = call "CardChannel2MuxChannel.vi"("Probecard Channel No."=w567) -> ("Mux No. string"=w568:string, "C1 / C2"=w569:i32, "Channel"=w566:i32)  [unwired: 1 out]
                n301 = Search 1D Array(1D array=w564, element=w567) -> (index of element=w595:i32)  [unwired: 1 in]
                n302 = Decrement(x=w569) -> (x-1=w570:i32)
                n303 = Decrement(x=w566) -> (x-1=w588:i32)
                n304 = local read "Compliance exceeded"() -> (w583:bool)
                n305 = Equal?(x="MUX1", y=w568) -> (x = y?=w574:bool)
                n306 = Unbundle By Name(w578) -> ("SMU"=w577:refnum<class "SupplyControl.lvclass">)
                n307 = call-dynamic "Supply_ComplianceCheck.vi"("error in (no error)"=w580, "SupplyControl in"=w577) -> ("error out"=w600:errorcluster, "Compliance exceeded?"=w582:bool, "SupplyControl out"=w579:refnum<class "SupplyControl.lvclass">)  [unwired: 6 in, 1 out]
                n308 = local read "Current Threshold [nA]"() -> (w596:dbl)
                n309 = Select(t=0, s=w574, f=2) -> (s? t:f=w571:i32)
                n310 = local read "Display MUX"() -> (w587:bool[][])
                n311 = Add(x=w571, y=w570) -> (x+y=w565:i32)
                n312 = Or(x=w582, y=w583) -> (x .or. y?=w581:bool)
                n313 = call-dynamic "Supply_ReadCurrent.vi"("error in (no error)"=w600, "SupplyControl in"=w579) -> ("error out"=w576:errorcluster, "Current in nA"=w597:dbl)  [unwired: 7 in, 1 out]
                n314 = local read "Current Array IN [nA]"() -> (w594:dbl[])
                n315 = Index Array(array=w587, index (row)=w588, index (col)=w565) -> (element=w589:bool)
                n316 = local write "Compliance exceeded"(w581) -> ()
                n317 = Absolute Value(x=w597) -> (abs(x)=w593:dbl)
                n318 = Greater?(x=w593, y=w596) -> (0:w598:bool)
                n319 = Not(x=w589) -> (.not. x?=w585:bool)
                n320 = Less Than 0?(x=w595) -> (x < 0?=w586:bool)
                n321 = Not(x=w582) -> (.not. x?=w599:bool)
                n322 = Decrement(x=w567) -> (x-1=w591:i32)
                n323 = And(x=w586, y=w585) -> (x .and. y?=w584:bool)
                n324 = And(x=w599, y=w598) -> (x .and. y?=w590:bool)
                n325 = case shown="True" w584 {
                  tunnel: w593 -> [_ w607]
                  tunnel: w594 -> [w601 w606]
                  tunnel: [w601 w605] -> w592
                  tunnel: w591 -> [_ w602]
                  tunnel: w582 -> [_ w604]
                  tunnel: w590 -> [_ w603]
                  frame False {
                  }
                  frame True {
                    n326 = case shown="True" w603 {
                      tunnel: w602 -> [_ w611]
                      frame False {
                      }
                      frame True {
                        n327 = Increment(x=w611) -> (x+1=w610:i32)
                        n328 = local read "disabled channels IN"() -> (w612:i32[])
                        n329 = local read "Pinhole Flag"() -> (w608:i32)
                        n330 = local read "Flag IN"() -> (w614:i32[])
                        n331 = Replace Array Subset(array=w614, new element=w608, index=w611) -> (w613:i32[])
                        n332 = Build Array (concatenate)(w612, w610) -> (w609:i32[])
                        n333 = local write "Flag IN"(w613) -> ()
                        n334 = local write "disabled channels IN"(w609) -> ()
                      }
                    }
                    n335 = case shown="True" w604 {
                      tunnel: w602 -> [_ w615]
                      frame False {
                      }
                      frame True {
                        n336 = Increment(x=w615) -> (x+1=w616:i32)
                        n337 = local read "Flag IN"() -> (w620:i32[])
                        n338 = local read "disabled channels IN"() -> (w618:i32[])
                        n339 = Replace Array Subset(array=w620, new element=3, index=w615) -> (w619:i32[])
                        n340 = local write "Flag IN"(w619) -> ()
                        n341 = Build Array (concatenate)(w618, w616) -> (w617:i32[])
                        n342 = local write "disabled channels IN"(w617) -> ()
                      }
                    }
                    n343 = Replace Array Subset(array=w606, new element=w607, index=w602) -> (w605:dbl[])
                  }
                }
                n344 = local write "Current Array IN [nA]"(w592) -> ()
              }
              frame #2 {
                n345 = global read "InstrumentSetup.vi" "MUX & Matrix Configurations"() -> (w624:T2)
                n346 = Unbundle By Name(w624) -> ("Switching"=w623:refnum<class "Switching.lvclass">, "Matrix X Channels.Mux2 C2"=w622:i32)
                n347 = stacked-sequence {
                  seq-local: [w632 _ _] -> [_ w639 _]
                  tunnel: w626 -> [w631 _ _]
                  tunnel: w628 -> [_ w640 _]
                  tunnel: [_ w638 _] -> w625
                  tunnel: w627 -> [_ _ w647]
                  tunnel: w623 -> [w629 w637 _]
                  tunnel: w622 -> [w630 w636 _]
                  frame #0 {
                    w633 = u16 0 items=["Open", "Close"] ("Switch action")
                    n348 = call "MatrixSwitchSingle.vi"("Switch action"=w633, "error in (no error)"=w631, "Matrix Y"=2, "Matrix X"=w630, "Switching in"=w629) -> ("error out"=w632:errorcluster)  [unwired: 4 in, 2 out]
                  }
                  frame #1 {
                    n349 = local read "disabled channels IN"() -> (w635:i32[])
                    n350 = Search 1D Array(1D array=w635, element=w640) -> (index of element=w642:i32)  [unwired: 1 in]
                    n351 = Less Than 0?(x=w642) -> (x < 0?=w643:bool)
                    n352 = case shown="True" w643 {
                      tunnel: [w645 w646] -> w641
                      frame False {
                        w645 = u16 0 items=["Open", "Close"] ("Switch action")
                      }
                      frame True {
                        w646 = u16 1 items=["Open", "Close"] ("Switch action")
                      }
                    }
                    n353 = call "MatrixSwitchSingle.vi"("Switch action"=w641, "error in (no error)"=w639, "Matrix Y"=1, "Matrix X"=w636, "Switching in"=w637) -> ("error out"=w638:errorcluster)  [unwired: 4 in, 2 out]
                  }
                  frame #2 {
                    n354 = Wait (ms)(milliseconds to wait=w647) -> ()  [unwired: 1 out]
                  }
                }
              }
              frame #3 {
                n355 = stacked-sequence {
                  seq-local: [w658 _] -> [_ w669]
                  tunnel: w653 -> [w659 _]
                  tunnel: w650 -> [w657 _]
                  tunnel: [w654 _] -> w649
                  tunnel: [_ w669] -> w652
                  tunnel: w651 -> [_ w668]
                  frame #0 {
                    n356 = global read "InstrumentSetup.vi" "MUX & Matrix Configurations"() -> (w656:T2)
                    n357 = Less?(x=w659, y=8) -> (x < y?=w661:bool)
                    n358 = case shown="True" w661 {
                      tunnel: w659 -> [w665 w667]
                      tunnel: [w665 w666] -> w658
                      frame False {
                      }
                      frame True {
                        n359 = Increment(x=w667) -> (x+1=w666:i32)
                      }
                    }
                    n360 = Unbundle By Name(w656) -> ("Switching"=w655:refnum<class "Switching.lvclass">)
                    n361 = call "CardChannel2MuxChannel.vi"("Probecard Channel No."=w658) -> ("Mux No.:"=w662:u32, "C1 / C2"=w663:i32, "Channel"=w664:i32)  [unwired: 1 out]
                    n362 = call "MuxSwitchSingle.vi"("MUX address"=w662, "error in (no error)"=w657, "Channel"=w664, "C1 / C2"=w663, "Switching in"=w655) -> ("error out"=w654:errorcluster)  [unwired: 4 in, 2 out]
                  }
                  frame #1 {
                    n363 = Wait (ms)(milliseconds to wait=w668) -> ()  [unwired: 1 out]
                  }
                }
                n364 = local read "Display MUX"() -> (w648:bool[][])
              }
            }
          }
        }
        n365 = And Array Elements(Boolean array=w42) -> (logical AND=w41:bool)
      }
      "Flag OUT" <- w33
      "Current Array OUT [nA]" <- w32
      "disabled channels OUT" <- w31
    }
  }
